vi "Avantes - AVS_GetSaturatedPixels.vi"(8 "error in (no error)":errorcluster, 11 "Cluster in":T1) -> (0 "error out":errorcluster, 1 "a_pSaturated":u8[](array[numeric]), 2 "Saturated?":bool, 3 "Cluster out":T1)   [LabVIEW 2013, in "Avantes Spectrometer Functions.lvlib"]
uses:
  Avantes Spectrometer Functions.lvlib
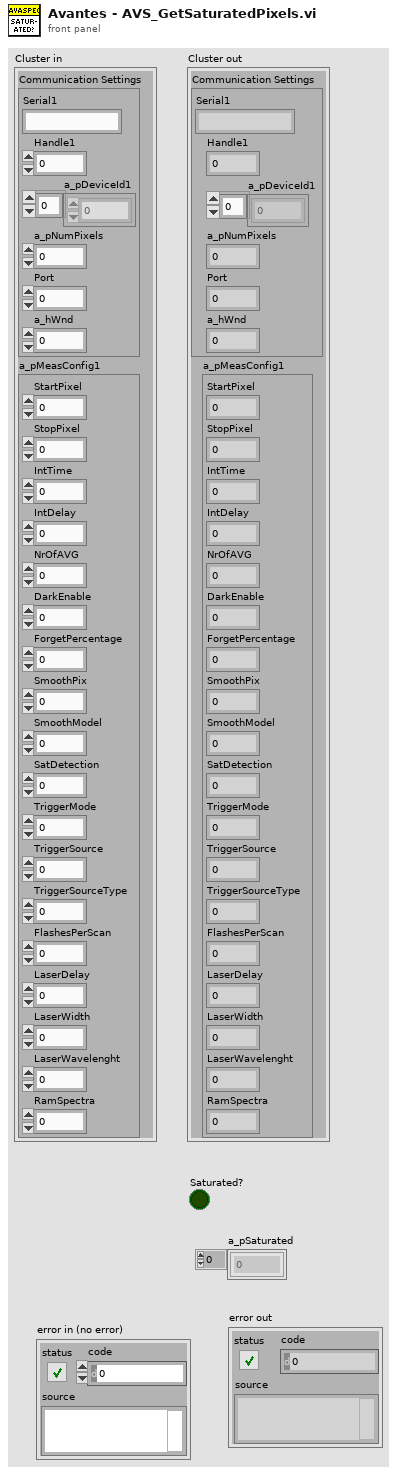
[diagram p1: front panel]
types:
  T1 = cluster{"Communication Settings":cluster{"Serial1":string, "Handle1":i32, "a_pDeviceId1":u8[], "a_pNumPixels":u16, "Port":i32, "a_hWnd":i32}, "a_pMeasConfig1":cluster{"StartPixel":u16, "StopPixel":u16, "IntTime":sgl, "IntDelay":u32, "NrOfAVG":u32, "DarkEnable":u8, "ForgetPercentage":u8, "SmoothPix":u16, "SmoothModel":u8, "SatDetection":u8, "TriggerMode":u8, "TriggerSource":u8, "TriggerSourceType":u8, "FlashesPerScan":u16, "LaserDelay":u32, "LaserWidth":u32, "LaserWavelenght":sgl, "RamSpectra":u16}}
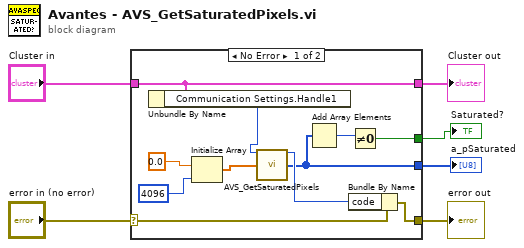
[diagram p0: block diagram]
diagram:
  n1 = case shown="No Error" "error in (no error)" {
    selector: "error in (no error)" -> [w16 w19]
    tunnel: [w17 w18] -> w6
    tunnel: "Cluster in" -> [w17 w18]
    tunnel: [w15 w19] -> w3
    tunnel: [w9 _] -> w2
    tunnel: [w7 _] -> w1
    frame No Error {
      n2 = Unbundle By Name(w17) -> ("Communication Settings.Handle1"=w13:i32)
      n3 = Initialize Array(0.0 ("element"), 4096 ("dimension size")) -> (w10:dbl[])
      n4 = call "AVS_GetSaturatedPixels.vi"("a_hDevice"=w13, "a_pSaturated"=w10) -> ("Output Value"=w14:i32, "a_pSaturated"=w9:u8[])  [unwired: 12 in]
      n5 = Add Array Elements(numeric array=w9) -> (sum=w8:u8)
      n6 = Bundle By Name(cluster=w16, "code"=w14) -> (w15:errorcluster)
      n7 = Not Equal To 0?(x=w8) -> (x != 0?=w7:bool)
    }
    frame Error {
    }
  }
  "Cluster out" <- w6
  "error out" <- w3
  "a_pSaturated" <- w2
  "Saturated?" <- w1
